vi "RampScript.vi"() -> ()   [LabVIEW 2017]
uses:
  FrontPanelReferences.vi
  Desktop/AODExperimentControls/ImageAcquisitionProgram/ImageAcquisitionLibrary/GlobalFrontPanelReferences.vi
  Desktop/AODExperimentControls/ImageAcquisitionProgram/ImageAcquisitionLibrary/ImageAcquisitionLibrary.lvlib
panel:
  in  "Relax Time":u32=1000
  in  "Record Time":u32=15000
  in  "B_f^2":dbl
  in  "B_0^2":dbl
  in  "Steps":i32=30
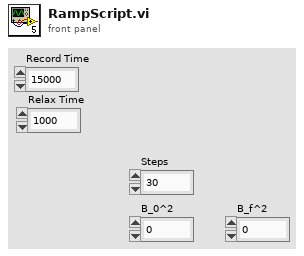
[diagram p1: front panel]
types:
  T1 = typedef "ImageAcquisitionLibrary.lvlib/References.ctl" = cluster{"Acquire":refnum<vi>, "Rec":refnum<vi>, "Tracking":refnum<vi>, "Settings":refnum<vi>, "Stop":refnum<vi>, "Initialized?":bool, "ImDisplay":refnum<vi>}
  T2 = typedef "WaveformGenerator.lvlib/WaveformGeneratorInterfaceRef.ctl" = cluster{"Waveform X":refnum<vi>, "Waveform Y":refnum<vi>, "Waveform Z":refnum<vi>, "Amplitude X":refnum<vi>, "Amplitude Y":refnum<vi>, "Amplitude Z":refnum<vi>, "Frequency X":refnum<vi>, "Frequency Y":refnum<vi>, "Frequency Z":refnum<vi>, "Phase X":refnum<vi>, "Phase Y":refnum<vi>, "Phase Z":refnum<vi>, "Offset X":refnum<vi>, "Offset Y":refnum<vi>, "Offset Z":refnum<vi>, "Stop":refnum<vi>, "On/Off":refnum<vi>, "Field^2":refnum<vi>}
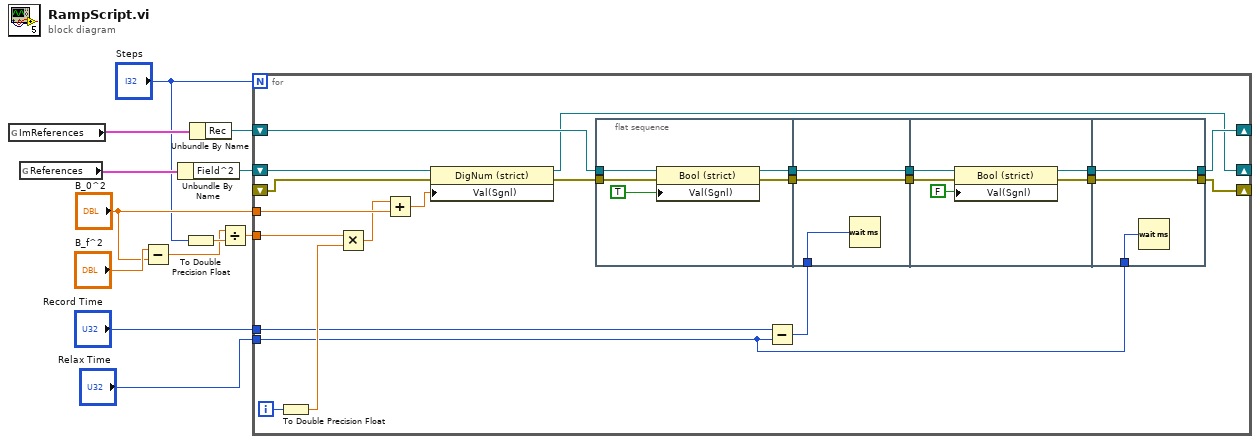
[diagram p0: block diagram]
diagram:
  n1 = global read "GlobalFrontPanelReferences.vi" "ImReferences"() -> (w10:T1)
  n2 = global read "FrontPanelReferences.vi" "References"() -> (w12:T2)
  n3 = Subtract(x="B_f^2", y="B_0^2") -> (x-y=w5:dbl)
  n4 = Unbundle By Name(w12) -> ("Field^2"=w11:refnum<vi>)
  n5 = To Double Precision Float(number="Steps") -> (double precision float=w6:dbl)
  n6 = Unbundle By Name(w10) -> ("Rec"=w3:refnum<vi>)
  n7 = Divide(x=w5, y=w6) -> (x/y=w4:dbl)
  n8 = for {
    N: "Steps" -> [_]
    shift-right: [w20] -> _
    shift-left: w3 -> [w19]
    shift-right: [w16] -> _
    shift-left: w11 -> [w33]
    shift-right: [w17] -> _
    shift-left: _ -> [w32]
    tunnel: "B_0^2" -> [w31]
    tunnel: w4 -> [w29]
    tunnel: "Record Time" -> [w15]
    tunnel: "Relax Time" -> [w13]
    i -> [w34]
    n9 = To Double Precision Float(number=w34) -> (double precision float=w30:dbl)
    n10 = Multiply(x=w29, y=w30) -> (x*y=w28:dbl)
    n11 = Add(x=w28, y=w31) -> (x+y=w27:dbl)
    n12 = property class="DigNum (strict)"(reference=w33, error in=w32, "Val(Sgnl)"=w27) -> (reference out=w16:refnum<vi>, error out=w26:errorcluster)
    n13 = flat-sequence {
      tunnel: w19 -> [w39]
      tunnel: w26 -> [w38]
      tunnel: [w37] -> w25
      tunnel: [w36] -> w24
      tunnel: w25 -> [w42]
      tunnel: w24 -> [w41]
      tunnel: [w42] -> w23
      tunnel: [w41] -> w22
      tunnel: w14 -> [w40]
      tunnel: w23 -> [w47]
      tunnel: w22 -> [w46]
      tunnel: [w44] -> w21
      tunnel: [w43] -> w18
      tunnel: [w50] -> w20
      tunnel: w21 -> [w50]
      tunnel: [w49] -> w17
      tunnel: w18 -> [w49]
      tunnel: w13 -> [w48]
      frame #0 {
        n14 = property class="Bool (strict)"(reference=w39, error in=w38, "Val(Sgnl)"=TRUE) -> (reference out=w37:refnum<vi>, error out=w36:errorcluster)
      }
      frame #1 {
        n15 = Wait (ms)(milliseconds to wait=w40) -> ()  [unwired: 1 out]
      }
      frame #2 {
        n16 = property class="Bool (strict)"(reference=w47, error in=w46, "Val(Sgnl)"=FALSE) -> (reference out=w44:refnum<vi>, error out=w43:errorcluster)
      }
      frame #3 {
        n17 = Wait (ms)(milliseconds to wait=w48) -> ()  [unwired: 1 out]
      }
    }
    n18 = Subtract(x=w15, y=w13) -> (x-y=w14:u32)
  }
